vi "FPGA Ref Manager.vi"(6 "Action":T2, 7 "error in (no error)":errorcluster, 10 "Generic FPGA Reference in":T1) -> (0 "error out":errorcluster, 3 "Generic FPGA Reference out":T1)   [LabVIEW 2021]
uses:
  <vilib>/myRIO/Common/Instrument Driver Framework/Utilities/typedefs/FPGA Ref Manager Action Enum.ctl
  <vilib>/myRIO/Common/Instrument Driver Framework/Utilities/typedefs/Generic FPGA Reference.ctl
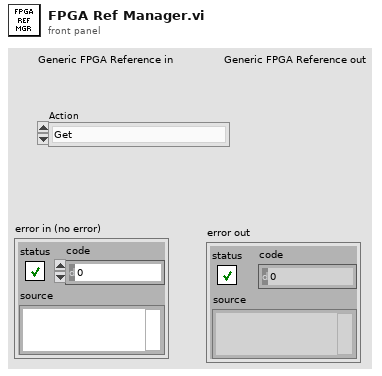
[diagram p1: front panel]
types:
  T1 = typedef "Generic FPGA Reference.ctl" = refnum<k20>
  T2 = typedef "FPGA Ref Manager Action Enum.ctl" = enum16{"Get", "Set", "Reset"}
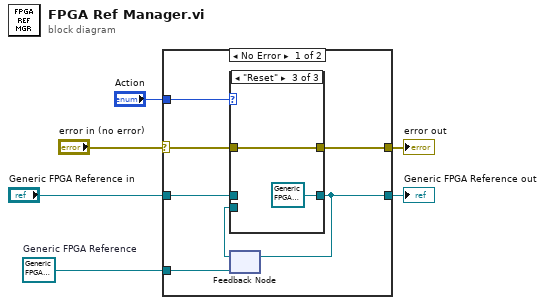
[diagram p0: block diagram]
diagram:
  w4 = T1 refnum  # Generic FPGA Reference
  n1 = case shown="No Error" "error in (no error)" {
    selector: "error in (no error)" -> [w8 w20]
    tunnel: "Action" -> [w12 _]
    tunnel: "Generic FPGA Reference in" -> [w11 _]
    tunnel: w4 -> [w10 w21]
    tunnel: [w9 w20] -> w3
    tunnel: [w7 w21] -> w2
    frame No Error {
      n2 = feedback #1(w10) -> (w13:T1)
      n3 = case shown="\"Reset\"" w12 {
        tunnel: [w14 w16 T1 refnum ("Generic FPGA Reference in")] -> w7
        tunnel: w13 -> [_ w16 _]
        tunnel: w11 -> [w14 _ _]
        tunnel: w8 -> [w15 w17 w19]
        tunnel: [w15 w17 w19] -> w9
        frame "Set" {
        }
        frame "Get" {
        }
        frame "Reset" {
        }
      }
      n4 = feedback-in #1(w7) -> ()
    }
    frame Error {
    }
  }
  "Generic FPGA Reference out" <- w2
  "error out" <- w3
